vi "buildStartCycle.vi"(8 "error in (no error)":errorcluster, 11 "PlainTextCommandBuilder in":refnum<class "XMLCommandBuilder.lvclass">) -> (0 "error out":errorcluster, 2 "message":string, 3 "PlainTextCommandBuilder out":refnum<class "XMLCommandBuilder.lvclass">)   [LabVIEW 2023, in "AbstractFactory.lvlib" / "XMLCommandBuilder.lvclass"]
uses:
  XMLCommandBuilder.lvclass
  XMLCommandBuilder.lvclass/XMLCommandBuilder.ctl
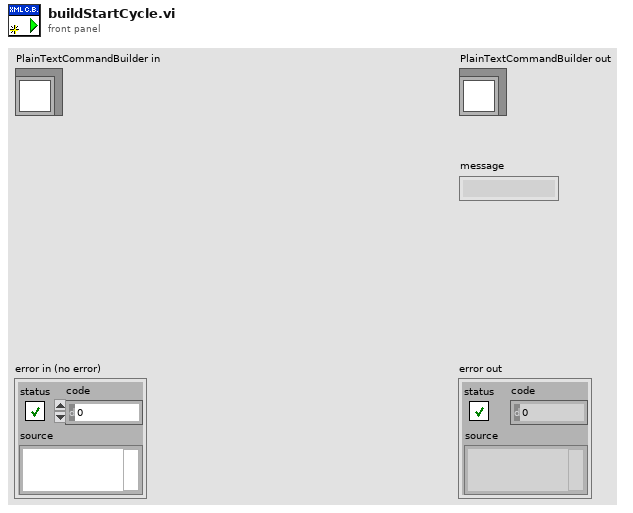
[diagram p1: front panel]
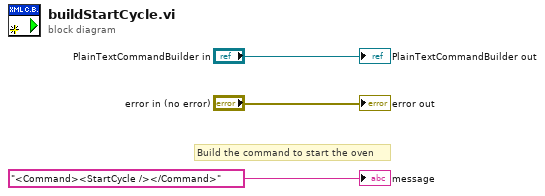
[diagram p0: block diagram]
diagram:
  # "Build the command to start the oven"
  "error out" <- "error in (no error)"
  "PlainTextCommandBuilder out" <- "PlainTextCommandBuilder in"
  "message" <- "<Command><StartCycle /></Command>" ("message")
